vi "利用变体做字典容器.vi"() -> ()   [LabVIEW 2009]
panel:
  out "学生成绩":dbl
  in  "查询姓名":string
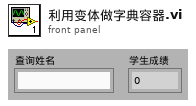
[diagram p1: front panel]
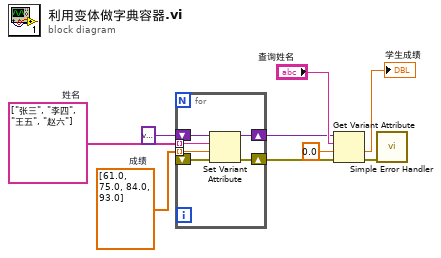
[diagram p0: block diagram]
diagram:
  w7 = dbl[] [61.0, 75.0, 84.0, 93.0]  # 成绩
  w8 = string[] ["张三", "李四", "王五", "赵六"]  # 姓名
  n1 = for {
    shift-right: [w12] -> w4
    shift-left: variant ("variant") -> [w15]
    tunnel: w8 -> [w14] mode=indexing
    tunnel: w7 -> [w13] mode=indexing
    shift-right: [w10] -> w2
    shift-left: _ -> [w11]
    n2 = Set Variant Attribute(Variant=w15, name=w14, value=w13, error in=w11) -> (Variant out=w12:variant, error out=w10:errorcluster)  [unwired: 1 out]
  }
  n3 = Get Variant Attribute(Variant=w4, name="查询姓名", default value (empty Variant)=0.0, error in=w2) -> (value=→"学生成绩":dbl, error out=w1:errorcluster)  [unwired: 2 out]
  n4 = call <vilib>:"Simple Error Handler.vi"("error in (no error)"=w1) -> ()  [unwired: 4 in, 5 out]
